vi "Stereo - Analyze Grid Coverage.vi"(8 "error in (no error)":errorcluster, 9 "Coverage Threshold %":dbl=75.0, 10 "# of Zones":i32=3, 11 "Grid Coverage":T2) -> (0 "error out":errorcluster, 1 "Coverage %":string[][](array[string]), 2 "Quadrants OK":bool[][](array[boolean]), 3 "Grid Coverage (dup)":T2, 4 "Coverage OK":bool)   [LabVIEW 2019]
doc: "Analyse each quadrant of the image to verify if at least one quadrant is 80% covered to insure proper single calibration."
uses:
  <vilib>/vision/Image Controls.llb/IMAQ Image.ctl
  <vilib>/vision/NI_Vision_Development_Module.lvlib
panel:
  in  "Coverage Index":T1(array[cluster])=[{"Coverage Index"=[{"Row (y)"=0, "Col (x)"=0}, {"Row (y)"=0, "Col (x)"=2}, {"Row (y)"=1, "Col (x)"=1}]}, {"Coverage Index"=[{"Row (y)"=0, "Col (x)"=2}, {"Row (y)"=2, "Col (x)"=2}, {"Row (y)"=1, "Col (x)"=1}]}, {"Coverage Index"=[{"Row (y)"=2, "Col (x)"=0}, {"Row (y)"=2, "Col (x)"=2}, {"Row (y)"=1, "Col (x)"=1}]}, {"Coverage Index"=[{"Row (y)"=0, "Col (x)"=0}, {"Row (y)"=2, "Col (x)"=0}, {"Row (y)"=1, "Col (x)"=1}]}]
  # "Overview: Analyse each quadrant of the image to verify if at least one quadrant is 80% covered to insure proper single calibration."
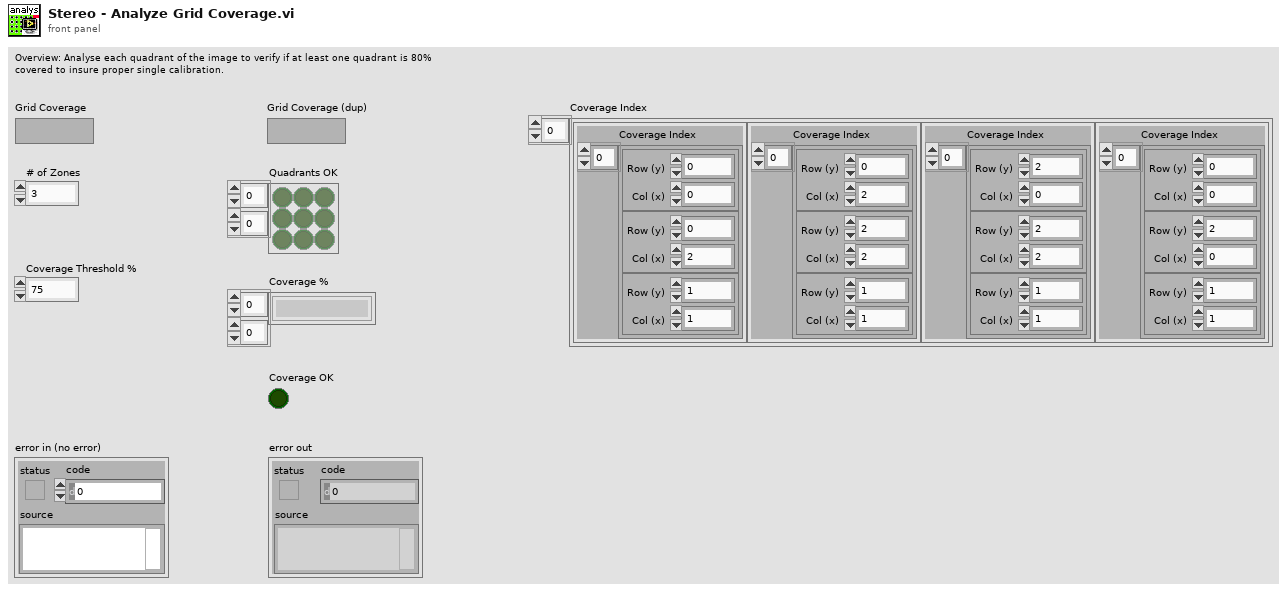
[diagram p1: front panel]
types:
  T1 = cluster{"Coverage Index":cluster{"Row (y)":i32, "Col (x)":i32}[]}[]
  T2 = typedef "IMAQ Image.ctl" = refnum<image>
  T3 = cluster{"histogram":u32[], "Minimal Value":sgl, "Maximal Value":sgl, "Starting Value":sgl, "Interval Width":sgl, "Mean Value":sgl, "Standard  Variation":sgl, "Area (pixels)":i32}
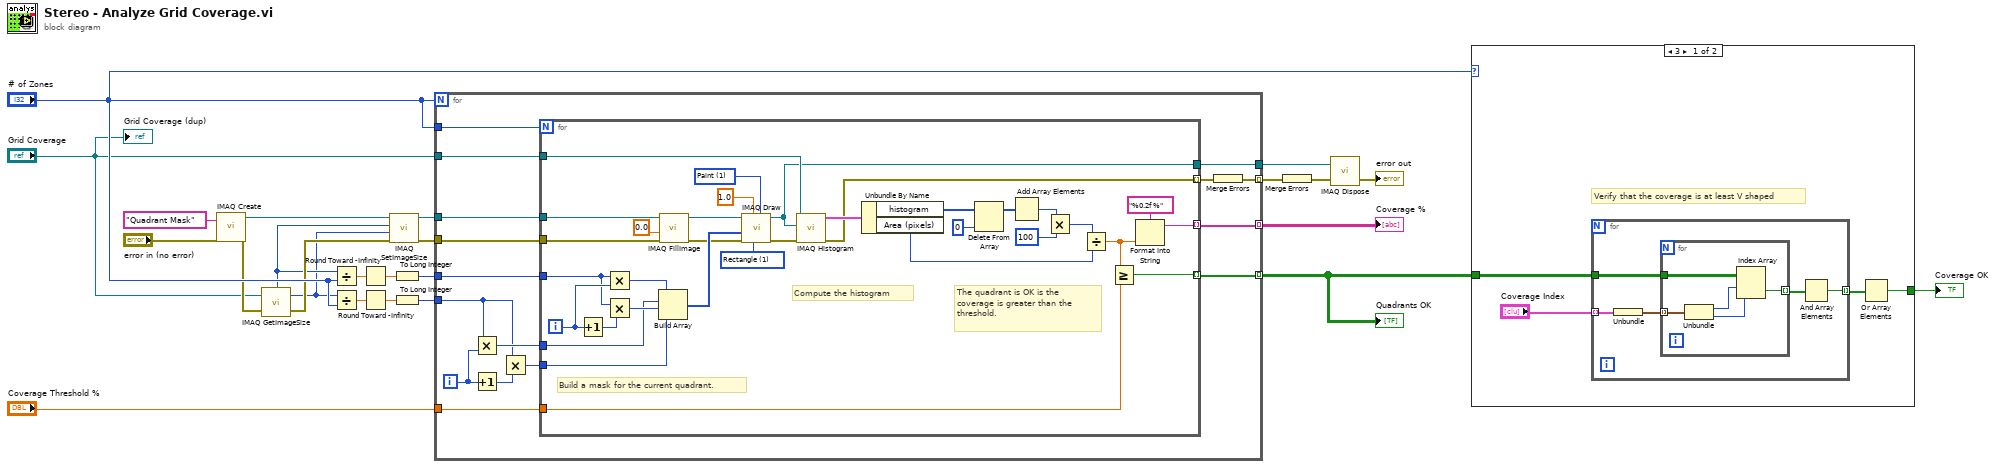
[diagram p0: block diagram]
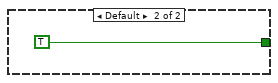
[diagram p2: hidden frame]
diagram:
  n1 = call "IMAQ Create"("Image Name"="Quadrant Mask", "error in (no error)"="error in (no error)") -> ("New Image"=w20:T2, "error out"=w19:errorcluster)  [unwired: 2 in, 1 out]
  n2 = call "IMAQ GetImageSize"("Image"="Grid Coverage", "error in (no error)"=w19) -> ("Y Resolution"=w6:i32, "X Resolution"=w7:i32, "error out"=w14:errorcluster)  [unwired: 2 out]
  n3 = Divide(x=w7, y="# of Zones") -> (x/y=w18:dbl)
  n4 = Divide(x=w6, y="# of Zones") -> (x/y=w17:dbl)
  n5 = Round Toward -Infinity(1:w18) -> (0:w16:dbl)
  n6 = Round Toward -Infinity(1:w17) -> (0:w15:dbl)
  n7 = call "IMAQ SetImageSize"("error in (no error)"=w14, "Y Resolution"=w6, "X Resolution"=w7, "Image"=w20) -> ("error out"=w3:errorcluster, "Image Out"=w12:T2)  [unwired: 1 out]
  n8 = To Long Integer(number=w16) -> (32bit integer=w11:i32)
  n9 = To Long Integer(number=w15) -> (32bit integer=w10:i32)
  n10 = for {
    N: "# of Zones" -> [_]
    tunnel: w12 -> [w37]
    tunnel: w11 -> [w36]
    tunnel: w10 -> [w31]
    tunnel: [w35] -> w24 mode=indexing
    tunnel: "Grid Coverage" -> [w34]
    tunnel: [w33] -> w8
    tunnel: "# of Zones" -> [w32]
    tunnel: [w30] -> w5 mode=indexing
    tunnel: "Coverage Threshold %" -> [w29]
    tunnel: w3 -> [w28]
    tunnel: [w26] -> w2 mode=indexing
    i -> [w39]
    n11 = Multiply(x=w31, y=w39) -> (x*y=w41:i32)
    n12 = Increment(x=w39) -> (x+1=w40:i32)
    n13 = Multiply(x=w31, y=w40) -> (x*y=w38:i32)
    n14 = for {
      N: w32 -> [_]
      tunnel: w41 -> [w65]
      tunnel: w38 -> [w64]
      tunnel: w37 -> [w72]
      tunnel: w36 -> [w69]
      tunnel: [w63] -> w35 mode=indexing
      tunnel: w34 -> [w71]
      tunnel: [w70] -> w33
      tunnel: [w45] -> w30 mode=indexing
      tunnel: w29 -> [w44]
      tunnel: w28 -> [w43]
      tunnel: [w42] -> w27 mode=indexing
      i -> [w74]
      w49 = u16 1 items=["Line", "Rectangle", "Oval"] ("Shape to draw")
      w48 = u16 1 items=["Frame", "Paint", "Invert Frame", "Invert Paint"] ("Draw Mode")
      # "The quadrant is OK is the coverage is greater than the threshold."
      # "Compute the histogram"
      # "Build a mask for the current quadrant."
      n15 = Increment(x=w74) -> (x+1=w73:i32)
      n16 = Multiply(x=w69, y=w74) -> (x*y=w67:i32)
      n17 = Multiply(x=w69, y=w73) -> (x*y=w66:i32)
      n18 = Build Array(w67, w65, w66, w64) -> (w68:i32[])
      n19 = call "IMAQ FillImage"("error in (no error)"=w43, "Pixel Value (U8, U16, I16, Float)"=sgl 0.0, "Image"=w72) -> ("error out"=w52:errorcluster, "Image Out"=w51:T2)  [unwired: 4 in, 3 out]
      n20 = call "IMAQ Draw"("Draw Mode"=w48, "Shape to draw"=w49, "Pixel Color"=sgl 1.0, "error in (no error)"=w52, "Coordinates"=w68, "Image Src"=w51) -> ("error out"=w54:errorcluster, "Image Dst Out"=w70:T2)  [unwired: 1 in, 3 out]
      n21 = call "IMAQ Histogram"("error in (no error)"=w54, "Image Mask"=w70, "Image"=w71) -> ("error out"=w42:errorcluster, "Histogram Report"=w55:T3)  [unwired: 2 in, 5 out]
      n22 = Unbundle By Name(w55) -> ("histogram"=w56:u32[], "Area (pixels)"=w62:i32)
      n23 = Delete From Array(array=w56, index=0) -> (array with subset deleted=w58:u32[])  [unwired: 1 in, 1 out]
      n24 = Add Array Elements(numeric array=w58) -> (sum=w61:u32)
      n25 = Multiply(x=w61, y=u32 100) -> (x*y=w59:u32)
      n26 = Divide(x=w59, y=w62) -> (x/y=w47:dbl)
      n27 = Greater Or Equal?(x=w47, y=w44) -> (x >= y?=w63:bool)
      n28 = Format Into String(format string="%0.2f %", w47) -> (resulting string=w45:string)  [unwired: 2 in, 1 out]
    }
    n29 = Merge Errors(w27) -> (w26:errorcluster)
  }
  "Quadrants OK" <- w24
  "Coverage %" <- w5
  n30 = Merge Errors(w2) -> (w1:errorcluster)
  n31 = call "IMAQ Dispose"("Image"=w8, "error in (no error)"=w1) -> ("error out"=→"error out":errorcluster)  [unwired: 1 in, 3 out]
  n32 = case shown="3" "# of Zones" {
    tunnel: w24 -> [w77 _]
    tunnel: [w75 TRUE] -> w23
    frame 3 {
      # "Verify that the coverage is at least V shaped"
      n33 = for {
        tunnel: "Coverage Index" -> [w83] mode=indexing
        tunnel: w77 -> [w82]
        tunnel: [w79] -> w76 mode=indexing
        n34 = Unbundle(w83) -> ("Coverage Index"=w81:cluster{"Row (y)":i32, "Col (x)":i32}[])
        n35 = for {
          tunnel: w82 -> [w88]
          tunnel: w81 -> [w87] mode=indexing
          tunnel: [w84] -> w80 mode=indexing
          n36 = Unbundle(w87) -> ("Row (y)"=w86:i32, "Col (x)"=w85:i32)
          n37 = Index Array(array=w88, index (row)=w86, index (col)=w85) -> (element=w84:bool)
        }
        n38 = And Array Elements(Boolean array=w80) -> (logical AND=w79:bool)
      }
      n39 = Or Array Elements(Boolean array=w76) -> (logical OR=w75:bool)
    }
    frame Default {
    }
  }
  "Coverage OK" <- w23
  "Grid Coverage (dup)" <- "Grid Coverage"
